vi "Action_2.vi"(1 "Time Since Latch":u32, 2 "Instruction String":string) -> (0 "Advance Trigger":bool)   [LabVIEW 2018]
uses:
  instructions.vi
  sensors.vi
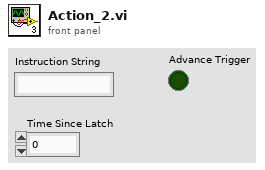
[diagram p1: front panel]
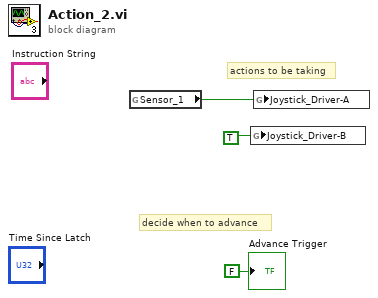
[diagram p0: block diagram]
diagram:
  # "actions to be taking"
  # "decide when to advance"
  n1 = global read "sensors.vi" "Sensor_1"() -> (w1:bool)
  n2 = global write "instructions.vi" "Joystick_Driver-B"(TRUE) -> ()
  n3 = global write "instructions.vi" "Joystick_Driver-A"(w1) -> ()
  "Advance Trigger" <- FALSE ("Advance Trigger")
